vi "Create Image Refs.vi"() -> (0 "error out":errorcluster, 1 "Template Report":T1={"Template Contrast"=0, "Grayvalue Max Pyramid Level"=-1, "Grayvalue Optimal Pyramid Level"=-1, "Gradient Max Pyramid Level"=-1, "Gradient Optimal Pyramid Level"=-1}, 2 "input cluster":T2)   [LabVIEW 2020]
uses:
  Type Defs/Image Refs.ctl
  <vilib>/vision/Image Controls.llb/IMAQ Image.ctl
  <vilib>/vision/NI_Vision_Development_Module.lvlib
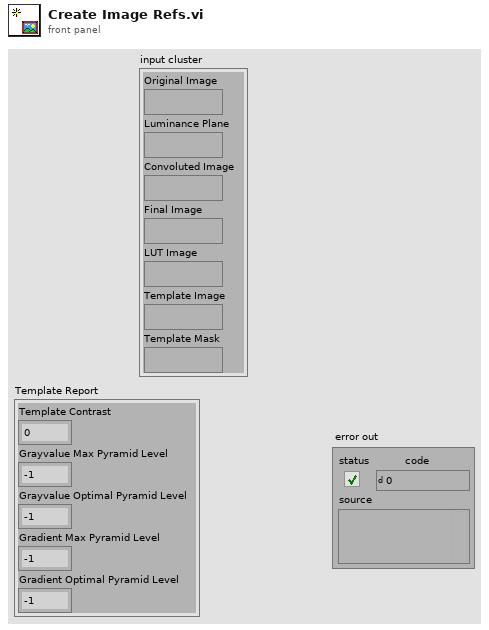
[diagram p1: front panel]
types:
  T1 = cluster{"Template Contrast":i32, "Grayvalue Max Pyramid Level":i32, "Grayvalue Optimal Pyramid Level":i32, "Gradient Max Pyramid Level":i32, "Gradient Optimal Pyramid Level":i32}
  T2 = typedef "Image Refs.ctl" = cluster{"Original Image":T3, "Luminance Plane":T3, "Convoluted Image":T3, "Final Image":T3, "LUT Image":T3, "Template Image":T3, "Template Mask":T3}
  T3 = typedef "IMAQ Image.ctl" = refnum<image>
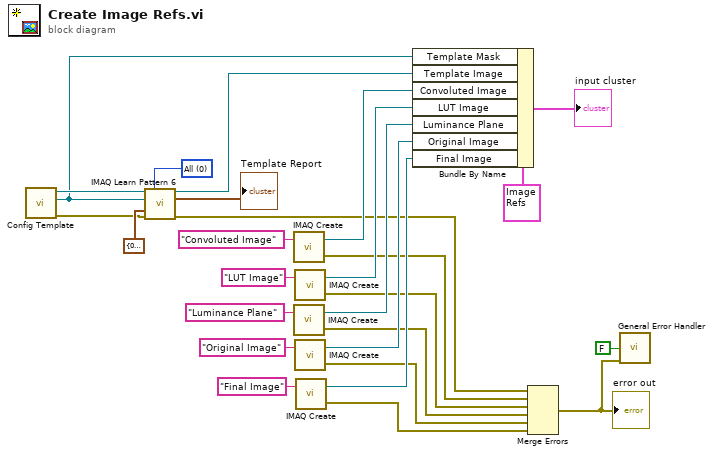
[diagram p0: block diagram]
diagram:
  w9 = 0 items=["All", "Low Discrepancy Sampling", "Grayscale Value Pyramid", "Gradients Pyramid"] ("Algorithm")
  n1 = call "Config Template.vi"() -> ("Template Image"=w3:T3, "Template Mask"=w1:T3, "error out"=w2:errorcluster)  [unwired: 1 in, 1 out]
  n2 = call "IMAQ Learn Pattern 6"("Image"=w3, "Algorithm"=w9, "Mask"=w1, "Angle Range"=cluster{"Start Angle":sgl, "End Angle":sgl} {"Start Angle"=0.0, "End Angle"=360.0}, "error in (no error)"=w2) -> ("Template Image Out"=w7:T3, "Template Report"=→"Template Report":T1, "error out"=w8:errorcluster)  [unwired: 8 in]
  n3 = call "IMAQ Create"("Image Name"="Convoluted Image") -> ("New Image"=w14:T3, "error out"=w12:errorcluster)  [unwired: 4 in]
  n4 = call "IMAQ Create"("Image Name"="Luminance Plane") -> ("New Image"=w24:T3, "error out"=w18:errorcluster)  [unwired: 4 in]
  n5 = call "IMAQ Create"("Image Name"="LUT Image") -> ("New Image"=w13:T3, "error out"=w11:errorcluster)  [unwired: 4 in]
  n6 = call "IMAQ Create"("Image Name"="Original Image") -> ("New Image"=w22:T3, "error out"=w17:errorcluster)  [unwired: 4 in]
  n7 = call "IMAQ Create"("Image Name"="Final Image") -> ("New Image"=w25:T3, "error out"=w16:errorcluster)  [unwired: 4 in]
  n8 = Bundle By Name(cluster=T2 {"Original Image"=refnum, "Luminance Plane"=refnum, "Convoluted Image"=refnum, "Final Image"=refnum, "LUT Image"=refnum, "Template Image"=refnum, "Template Mask"=refnum} ("input cluster"), "Template Mask"=w1, "Template Image"=w7, "Convoluted Image"=w14, "LUT Image"=w13, "Luminance Plane"=w24, "Original Image"=w22, "Final Image"=w25) -> (→"input cluster":T2)
  n9 = Merge Errors(w8, w12, w11, w18, w17, w16) -> (w5:errorcluster)
  "error out" <- w5
  n10 = call <vilib>:"General Error Handler.vi"("search ni.com link visible?(T)"=FALSE, "error in (no error)"=w5) -> ()  [unwired: 9 in, 5 out]
